vi "01 Controls and Indicators.vi"() -> ()   [LabVIEW 2020]
uses:
  _Subs/OpenDiagram/Open_XControl.xctl
panel:
  in  "OpenDiag":refnum<vi>(xcontrol)
  out "Gauge":dbl(knob) scale=0.0..10.0
  in  "Slide":dbl(slide)=5.204081632653061 scale=0.0..10.0
  # "01 Controls and Indicators\nThis code takes the value of the Slide and adds it to the Gauge\n\nInstructions:\n1. Hit the Run arrow and see the Gauge change to the value of the Slide\n2. Hit Continuous Run and watch the Gauge change as you vary the Slide"
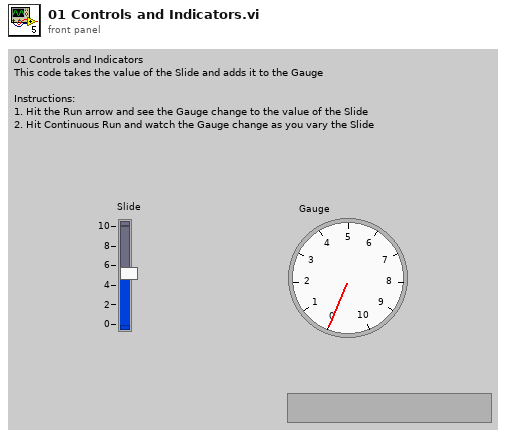
[diagram p1: front panel]
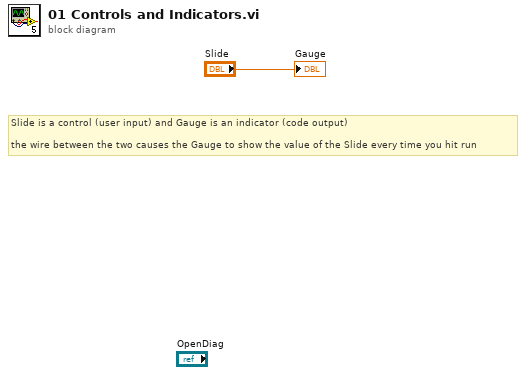
[diagram p0: block diagram]
diagram:
  # "Slide is a control (user input) and Gauge is an indicator (code output)\n\nthe wire between the two causes the Gauge to show the value of the Slide every time you hit run"
  "Gauge" <- "Slide"
